vi "TSM SSC Digital Filter Sites.vi"(0 "Digital TSM In":T1, 5 "Desired Sites":i32[](array[numeric]), 11 "error in":errorcluster) -> (4 "Digital TSM Out":T1, 15 "error out":errorcluster)   [LabVIEW 2019]
doc: "Use this VI to filter the Digital Cluster to contain only sessions and information pertaining to the desired sites. Note that the cluster information output by this function may be used for instrument control but should NOT be used to publish data to TSM."
uses:
  TSM SSC Digital.ctl
  <vilib>/NI_TestStand_SemiconductorModule/NI_TestStand_Semiconductor_Module.lvlibp/PinMap/Digital Pattern/PinQueryContext/DigitalPatternPinQueryContext.lvclass
  SSC Digital/SSC Digital.ctl
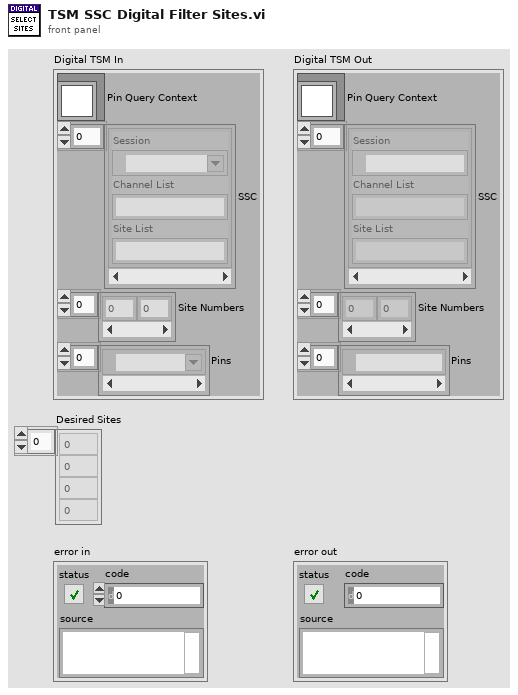
[diagram p1: front panel]
types:
  T1 = typedef "TSM SSC Digital.ctl" = cluster{"Pin Query Context":refnum<class "DigitalPatternPinQueryContext.lvclass">, "SSC":T2[], "Site Numbers":i32[], "Pins":tag[]}
  T2 = typedef "SSC Digital.ctl" = cluster{"Session":refnum<k15>, "Channel List":string, "Site List":string}
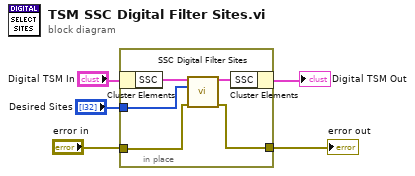
[diagram p0: block diagram]
diagram:
  n1 = in-place {
    in-place-border: "Desired Sites" -> [w10]
    in-place-border: "error in" -> [w7]
    in-place-border: [w6] -> w1
    n2 = in-place-cluster #1("Digital TSM In") -> ("SSC"=w9:T2[])
    n3 = call "SSC Digital Filter Sites.vi"("Digital SSC In"=w9, "Desired Sites"=w10, "error in"=w7) -> ("Digital SSC Out with requested sites"=w8:T2[], "error out"=w6:errorcluster)  [unwired: 11 in]
    n4 = in-place-cluster #1("SSC"=w8) -> (→"Digital TSM Out":T1)
  }
  "error out" <- w1
